vi "Apply Default.vi"(11 "Boolean in":refnum<class "Boolean.lvclass">) -> (3 "Boolean out":refnum<class "Boolean.lvclass">)   [LabVIEW 2020, in "Conditum.lvlib" / "Columns.lvlib" / "Boolean.lvclass"]
uses:
  Boolean.lvclass
  Boolean.lvclass/Boolean.ctl
  Type/Type.lvclass
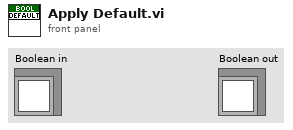
[diagram p1: front panel]
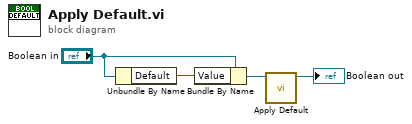
[diagram p0: block diagram]
diagram:
  n1 = Unbundle By Name("Boolean in") -> ("Default"=w3:bool)
  n2 = Bundle By Name(cluster="Boolean in", "Value"=w3) -> (w2:refnum<class "Boolean.lvclass">)
  n3 = call-parent "Apply Default.vi"("Type in"=w2) -> ("Type out"=→"Boolean out":refnum<class "Boolean.lvclass">)  [unwired: 10 in]
